vi "sumar numeros pares.vi"() -> ()   [LabVIEW 2020]
panel:
  out "Numeric 2":dbl
  out "Numeric":i32
  # "Programa que sume desde 0-10"
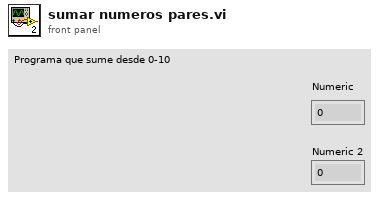
[diagram p1: front panel]
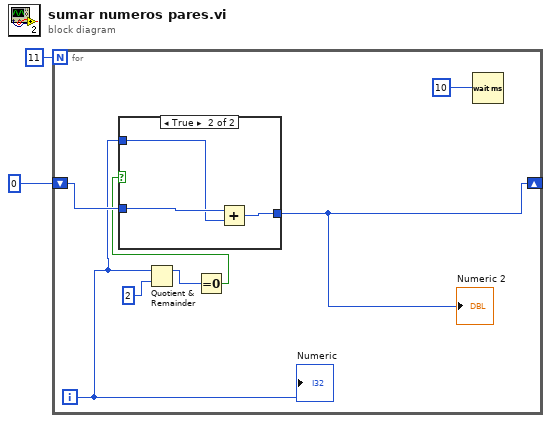
[diagram p0: block diagram]
diagram:
  n1 = for {
    N: 11 -> [_]
    shift-right: [w7] -> _
    shift-left: 0 -> [w8]
    i -> [w3]
    n2 = Quotient & Remainder(x=w3, y=2) -> (x-y*floor(x/y)=w5:i32)  [unwired: 1 out]
    n3 = Equal To 0?(x=w5) -> (x = 0?=w4:bool)
    n4 = case shown="True" w4 {
      tunnel: w8 -> [w10 w13]
      tunnel: [w10 w12] -> w7
      tunnel: w3 -> [_ w11]
      frame False {
      }
      frame True {
        n5 = Add(x=w13, y=w11) -> (x+y=w12:i32)
      }
    }
    "Numeric 2" <- w7
    n6 = Wait (ms)(milliseconds to wait=10) -> ()  [unwired: 1 out]
    "Numeric" <- w3
  }
